vi "Config_CheckGlobals.vi"(5 "GlobalsLED Ref":refnum<vi>, 7 "Status Ref":refnum<vi>, 8 "error in (no error)":errorcluster, 10 "Config Cluster":T2={"General"={"Config.ini"=path "", "Default Logging Path"=path ""}, "Hardware"={"Global T VAR"="", "Global B VAR"="", "VISAS"={"GEN COM"="", "SCOPE COM"="", "VNA COM"=""}}, "Operation"={"Operation Mode"=enum."Idle-Off", "Status"="", "NewLog?"=FALSE, "OvenWarn"=FALSE, "Scope Settings"={"TimeBase"=0.0, "VerticalScale"=4.0}}}, 11 "VISAS":T1) -> (0 "error out":errorcluster, 2 "Config Cluster Out":T2={"General"={"Config.ini"=path "", "Default Logging Path"=path ""}, "Hardware"={"Global T VAR"="", "Global B VAR"="", "VISAS"={"GEN COM"="", "SCOPE COM"="", "VNA COM"=""}}, "Operation"={"Operation Mode"=enum."Idle-Off", "Status"="", "NewLog?"=FALSE, "OvenWarn"=FALSE, "Scope Settings"={"TimeBase"=0.0, "VerticalScale"=4.0}}}, 3 "VISAS":T1)   [LabVIEW 2021]
uses:
  Config_Cluster.ctl
  Mode_Enum.ctl
  VISAS.ctl
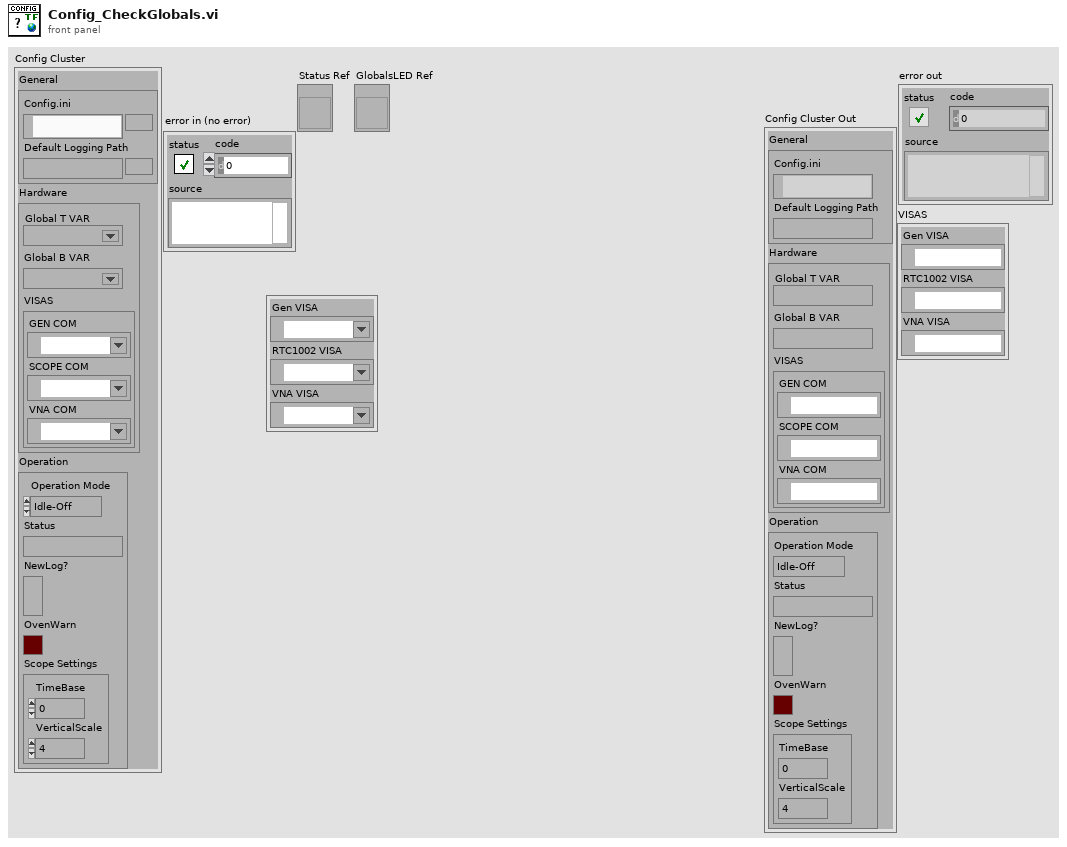
[diagram p1: front panel]
types:
  T1 = typedef "VISAS.ctl" = cluster{"Gen VISA":refnum<visa-resource-name>, "RTC1002 VISA":refnum<visa-resource-name>, "VNA VISA":refnum<visa-resource-name>}
  T2 = typedef "Config_Cluster.ctl" = cluster{"General":cluster{"Config.ini":path, "Default Logging Path":path}, "Hardware":cluster{"Global T VAR":refnum<k21>, "Global B VAR":refnum<k21>, "VISAS":cluster{"GEN COM":refnum<visa-resource-name>, "SCOPE COM":refnum<visa-resource-name>, "VNA COM":refnum<visa-resource-name>}}, "Operation":cluster{"Operation Mode":T3, "Status":string, "NewLog?":bool, "OvenWarn":bool, "Scope Settings":cluster{"TimeBase":dbl, "VerticalScale":dbl}}}
  T3 = typedef "Mode_Enum.ctl" = enum16{"OvenNRDY", "Logging", "Idle-Off", "Idle"}
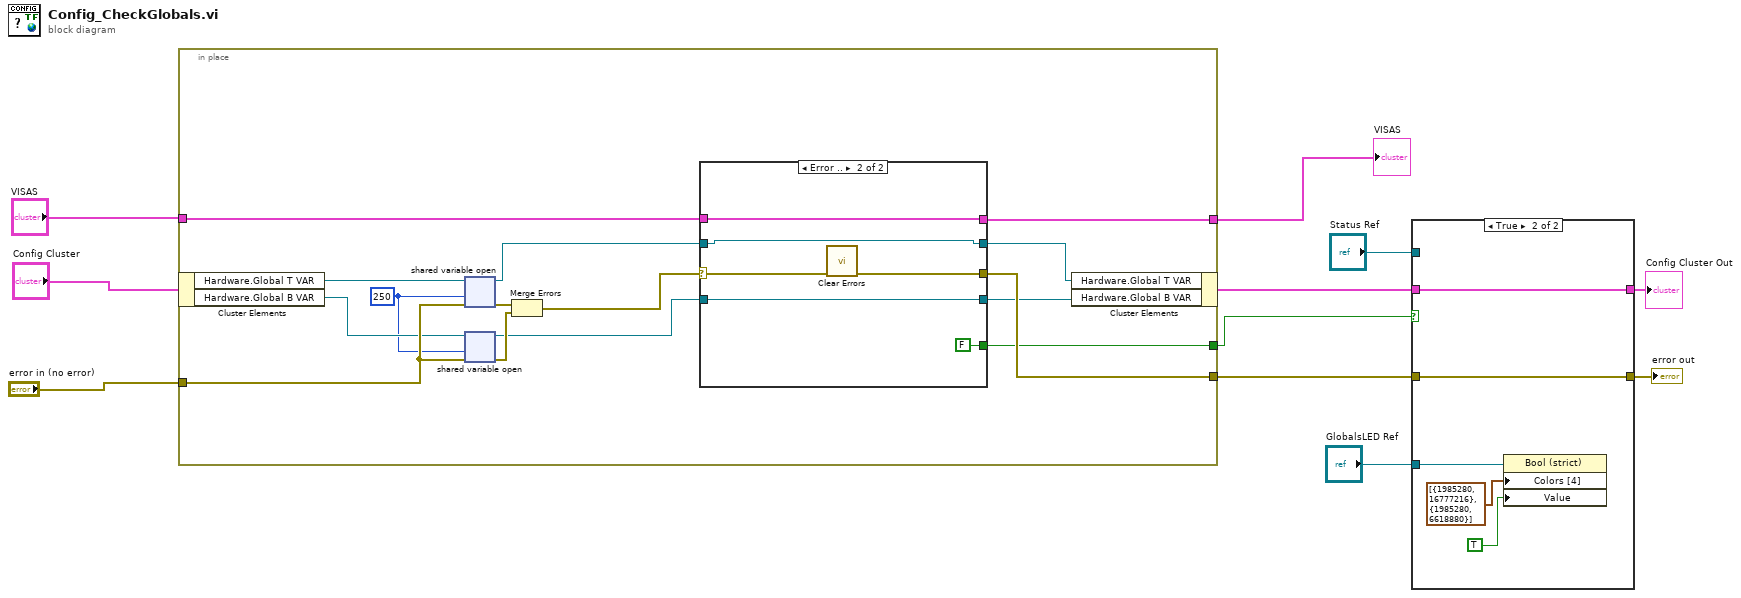
[diagram p0: block diagram]
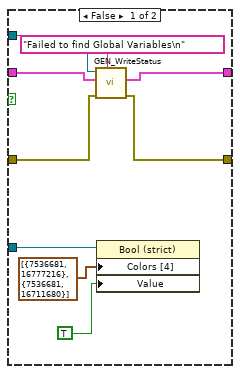
[diagram p2: hidden frame]
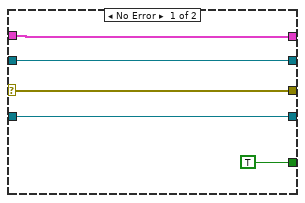
[diagram p3: hidden frame]
diagram:
  n1 = in-place {
    in-place-border: "VISAS" -> [w23]
    in-place-border: "error in (no error)" -> [w21]
    in-place-border: [w26] -> w1
    in-place-border: [w25] -> w6
    in-place-border: [w24] -> w8
    w19 = 250 ("timeout ms")
    n2 = in-place-cluster #1("Config Cluster") -> ("Hardware.Global T VAR"=w22:refnum<k21>, "Hardware.Global B VAR"=w20:refnum<k21>)
    n3 = shared-variable-open(w22, w21, w19) -> (w15:refnum<k21>, w18:errorcluster)  [unwired: 1 in]
    n4 = shared-variable-open(w20, w21, w19) -> (w14:refnum<k21>, w17:errorcluster)  [unwired: 1 in]
    n5 = Merge Errors(w18, w17) -> (w16:errorcluster)
    n6 = case shown="Error .." w16 {
      selector: w16 -> [w30 w36]
      tunnel: w23 -> [w31 w37]
      tunnel: [w31 w37] -> w26
      tunnel: [w30 w35] -> w25
      tunnel: [TRUE FALSE] -> w24
      tunnel: w15 -> [w28 w33]
      tunnel: w14 -> [w27 w32]
      tunnel: [w28 w33] -> w13
      tunnel: [w27 w32] -> w12
      frame No Error {
      }
      frame Error {
        n7 = call <vilib>:"Clear Errors.vi"("error in (no error)"=w36) -> ("error out"=w35:errorcluster)  [unwired: 5 in, 1 out]
      }
    }
    n8 = in-place-cluster #1("Hardware.Global T VAR"=w13, "Hardware.Global B VAR"=w12) -> (w9:T2)
  }
  "VISAS" <- w1
  n9 = case shown="True" w8 {
    tunnel: w9 -> [w46 w50]
    tunnel: "Status Ref" -> [w45 _]
    tunnel: w6 -> [w44 w51]
    tunnel: [w43 w51] -> w5
    tunnel: [w42 w50] -> w4
    tunnel: "GlobalsLED Ref" -> [w40 w49]
    frame False {
      n10 = call "GEN_WriteStatus.vi"("Input String"="Failed to find Global Variables\n", "error in (no error)"=w44, "Config_Cluster"=w46, "Status Ref"=w45) -> ("error out"=w43:errorcluster, "Config_Cluster Out"=w42:T2)  [unwired: 6 in]
      n11 = property class="Bool (strict)"(reference=w40, "Colors [4]"=cluster{u32, u32}[] [{7536681, 16777216}, {7536681, 16711680}], "Value"=TRUE) -> ()  [unwired: 1 in, 2 out]
    }
    frame True {
      n12 = property class="Bool (strict)"(reference=w49, "Colors [4]"=cluster{u32, u32}[] [{1985280, 16777216}, {1985280, 6618880}], "Value"=TRUE) -> ()  [unwired: 1 in, 2 out]
    }
  }
  "Config Cluster Out" <- w4
  "error out" <- w5
